vi "C4Dev_writeFile.vi"(0 "c4dev in":refnum<k24>, 5 "selector in":string, 7 "file path in":path, 11 "error in":errorcluster) -> (4 "c4dev out":refnum<k24>, 15 "error out":errorcluster)   [LabVIEW 2015, in "libC4HdlLV.lvlib"]
uses:
  libC4HdlLV.lvlib
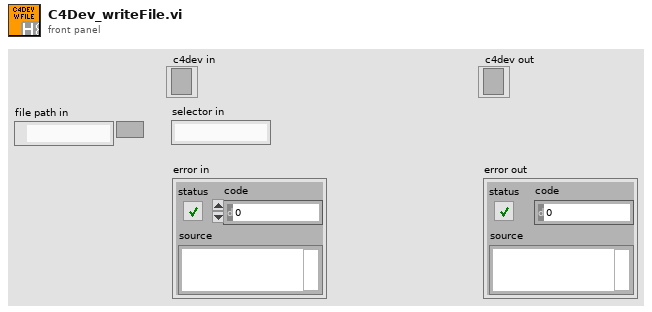
[diagram p1: front panel]
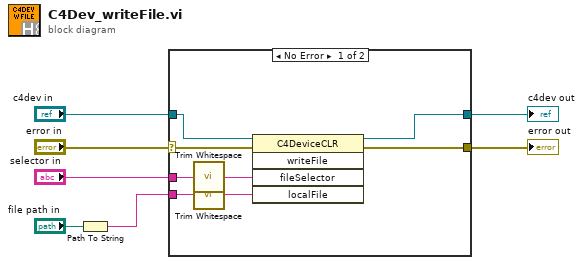
[diagram p0: block diagram]
diagram:
  n1 = Path To String(path="file path in") -> (string=w5:string)
  n2 = case shown="No Error" "error in" {
    selector: "error in" -> [w14 w17]
    tunnel: [w8 w16] -> w2
    tunnel: [w9 w17] -> w1
    tunnel: "selector in" -> [w15 _]
    tunnel: "c4dev in" -> [w13 w16]
    tunnel: w5 -> [w10 _]
    frame No Error {
      n3 = call <vilib>:"Trim Whitespace.vi"("string"=w15) -> ("trimmed string"=w12:string)  [unwired: 1 in]
      n4 = call <vilib>:"Trim Whitespace.vi"("string"=w10) -> ("trimmed string"=w11:string)  [unwired: 1 in]
      n5 = invoke class="C4DeviceCLR" method="writeFile"(reference=w13, error in=w14, "fileSelector"=w12, "localFile"=w11) -> (reference out=w8:refnum<k24>, error out=w9:errorcluster)  [unwired: 1 in, 3 out]
    }
    frame Error {
    }
  }
  "error out" <- w1
  "c4dev out" <- w2
